vi "New Game.vi"(0 "Display State In":T1={"method"=enum."None", "current color"=1, "available black position"=[], "available white position"=[], "Interactive Action"=refnum, "row"=0, "column"=0} caption="显示状态输入", 9 "Container State":T5 caption="容器状态", 11 "error in (no error)":errorcluster caption="错误输入（无错误）") -> (4 "Display State Out":T1={"method"=enum."None", "current color"=1, "available black position"=[], "available white position"=[], "Interactive Action"=refnum, "row"=0, "column"=0} caption="显示状态输出", 15 "error out":errorcluster caption="错误输出")   [LabVIEW 2018, in "Othello.xctl"]
doc: "本VI是为《我和LabVIEW》一书编写的示例。\n关于本书的介绍请参考网页：\nhttp://ruanqizhen.spaces.live.com/blog/cns!5852D4F797C53FB6!4310.entry"
uses:
  Othello.xctl
  Control/Method Call.ctl
  Control/Pict Ring Chess.ctl
  <vilib>/_xctls/Container State.ctl
  <vilib>/_xctls/XControlSupport.lvlib
  Ability/State.ctl
  Control/Interactive Action.ctl
types:
  T1 = typedef "Othello.xctl/State.ctl" = cluster{"method":T2, "current color":T3, "available black position":i32[][], "available white position":i32[][], "Interactive Action":T4, "row":i32, "column":i32}
  T2 = typedef "Othello.xctl/Method Call.ctl" = enum16{"None", "New Game", "Play One"}
  T3 = typedef "Othello.xctl/Pict Ring Chess.ctl" = u16
  T4 = typedef "Othello.xctl/Interactive Action.ctl" = refnum<user-event>
  T5 = typedef "XControlSupport.lvlib/Container State.ctl" = cluster{"Indicator?":bool, "Run Mode?":bool, " Refnum":refnum<vi>}
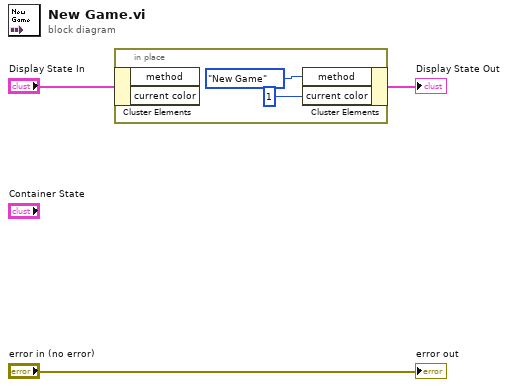
[diagram p0: block diagram]
diagram:
  n1 = in-place {
    n2 = in-place-cluster #1("Display State In") -> ()  [unwired: 2 out]
    n3 = in-place-cluster #1("method"=Method_Call."New Game", "current color"=T3 1) -> (→"Display State Out":T1)
  }
  "error out" <- "error in (no error)"
